vi "Generate D SIM IDs.vi"(1 "SIM FE (0=no sim)":u16 format="%016b", 2 "SIM PA (0=no sim)":u8 format="%08b", 3 "SIM RF (0=no sim)":u8 format="%08b") -> (0 "SIM ID":u32 format="%032b")   [LabVIEW 2011]
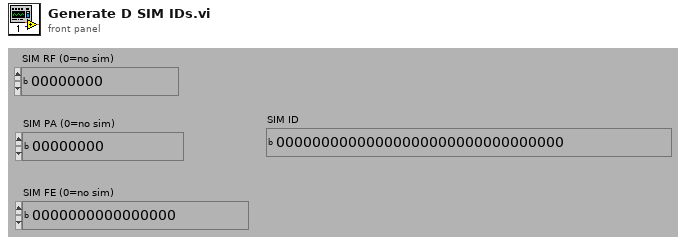
[diagram p1: front panel]
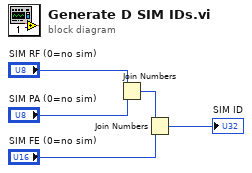
[diagram p0: block diagram]
diagram:
  n1 = Join Numbers(hi="SIM RF (0=no sim)", lo="SIM PA (0=no sim)") -> ((hi.lo)=w5:u16)
  n2 = Join Numbers(hi=w5, lo="SIM FE (0=no sim)") -> ((hi.lo)=→"SIM ID":u32)
